vi "Dashboard Main.vi"() -> ()   [LabVIEW 2017]
uses:
  <vilib>/Utility/miscctls.llb/LVRowAndColumnTypeDef.ctl
  <vilib>/event_ctls.llb/eventvkey.ctl
  <vilib>/Rock Robotics/Network Tables/NT Read Numeric Array.vi
  <vilib>/Rock Robotics/WPI/Dashboard/WPI_DashboardLogging Global.vi
panel:
  in  "Camera Settings Right":T1={"Frame Rate"=30, "Compression"=30, "Size"=1, "DB Camera Config"=FALSE} {"Frame Rate" scale=1.0..30.0; "Compression" scale=100.0..-1.0; "Size" items=["640x480", "320x240", "160x120"]}
  in  "Camera Name Right":string(combo)="No Camera Selection"
  out "Camera Info":cluster{"Mbps LED":bool, "Mbps":dbl, "fps":dbl} {"fps" format="%#.1g"; "Mbps" format="%#.1g"}
  in  "Camera Settings":T1={"Frame Rate"=30, "Compression"=30, "Size"=1, "DB Camera Config"=FALSE} {"Frame Rate" scale=1.0..30.0; "Compression" scale=100.0..-1.0; "Size" items=["640x480", "320x240", "160x120"]}
  in  "TCP":refnum<k5>
  in  "Rec Mode":enum32{"Stop", "Record", "Playback"}(radio)
  out "Robot IP":string
  out "Image Message":string="Timeout in Camera Communications"
  in  "Dashboard Tab":T2(tab)
  in  "Select Auto":string(combo)="Select Autonomous ..."
  out "NT Connection":bool
  out "MotorChart R":cluster{"Numeric":dbl, "Numeric":dbl}(graph)
  out "MotorChart L":cluster{"Numeric":dbl, "Numeric":dbl}(graph)
  out "MotorSliders R":cluster{"MotorSlide1":dbl, "MotorSlide2":dbl} {"MotorSlide2" scale=-1.0..1.0 scale format="%#_2e"; "MotorSlide1" scale=-1.0..1.0 scale format="%#_2e"}
  out "MotorSliders L":cluster{"MotorSlide1":dbl, "MotorSlide2":dbl} {"MotorSlide2" scale=-1.0..1.0 scale format="%#_2e"; "MotorSlide1" scale=-1.0..1.0 scale format="%#_2e"}
  out "Gyro":dbl(knob) scale=-360.0..360.0
  out "JS1 Z":dbl(slide) scale=-1.0..1.0 scale format="%#_2e"
  out "JS1 Graph":cluster{"X":dbl, "Y":dbl}[](graph)
  out "JS1 Buttons":T3
  out "JS2 Z":dbl(slide) scale=-1.0..1.0 scale format="%#_2e"
  out "JS2 Graph":cluster{"X":dbl, "Y":dbl}[](graph)
  out "JS2 Buttons":T3
  out "Mode":T4(ring)=enum."Auto Disabled"
  out "Left Position":dbl
  out "Right Position":dbl
  out "Camera Image Right":T5(plugin-control)
  in  "DB/String 9":string
  in  "DB/String 8":string
  in  "DB/String 7":string
  in  "DB/String 6":string
  in  "DB/String 5":string
  in  "DB/String 4":string
  in  "DB/String 3":string
  in  "DB/String 2":string
  in  "DB/String 1":string
  in  "DB/String 0":string
  in  "DB/Slider 0":dbl(slide) scale=0.0..5.0
  in  "DB/Slider 1":dbl(slide) scale=0.0..5.0
  in  "DB/Slider 2":dbl(slide) scale=0.0..5.0
  in  "DB/Slider 3":dbl(slide) scale=0.0..5.0
  out "DB/LED 3":bool
  out "DB/LED 2":bool
  out "DB/LED 1":bool
  out "DB/LED 0":bool
  in  "DB/Button 3":bool
  in  "DB/Button 2":bool
  in  "DB/Button 1":bool
  in  "DB/Button 0":bool caption="New Name"
  out "Tusk Left Output":dbl
  out "Game Specific Data":string
  out "DriveL Position":dbl
  out "DriveR Position":dbl
  out "Tusk Right Position":dbl
  out "Tusk Left Position":dbl
  out "Elbow Position":dbl
  out "Arm Position":dbl
  out "Tusk Right Output":dbl
  in  "Test Slider":dbl(slide) scale=0.0..100.0 scale format="%#_3g"
  in  "On/Off":bool caption="Solenoid"
  in  "Test Name":u16(ring) items=["Select the test to run..."]
  in  "Test Tree":string(tree)
  in  "Motor":cluster{"Value":dbl, "Enable":bool} {"Value" scale=-1.0..1.0 scale format="%#_3g"}
  out "Progress":T6 {"Test Progress" scale=0.0..100.0}
  in  "Rev/Fwd":cluster{"Forward":bool, "Reverse":bool}
  in  "Test Ring":u16(ring) items=["Monochrome", "Color"]
  out "Cmd Status":string
  in  "Execute Command":bool
  in  "Command Params":string[][](table)
  in  "Command Selection":i32(listbox)
  in  "CheckList":i32(listbox)
  out "Tree":string(tree)
  out "Camera Image":T5(plugin-control)
  out "Background":bool
  in  "Camera Name":string(combo)="No Camera Selection"
  # "HW"
  # "HW"
  # "Joysticks"
  # "Drive Motors"
  # "Front"
  # "Right"
  # "Left"
  # "Back"
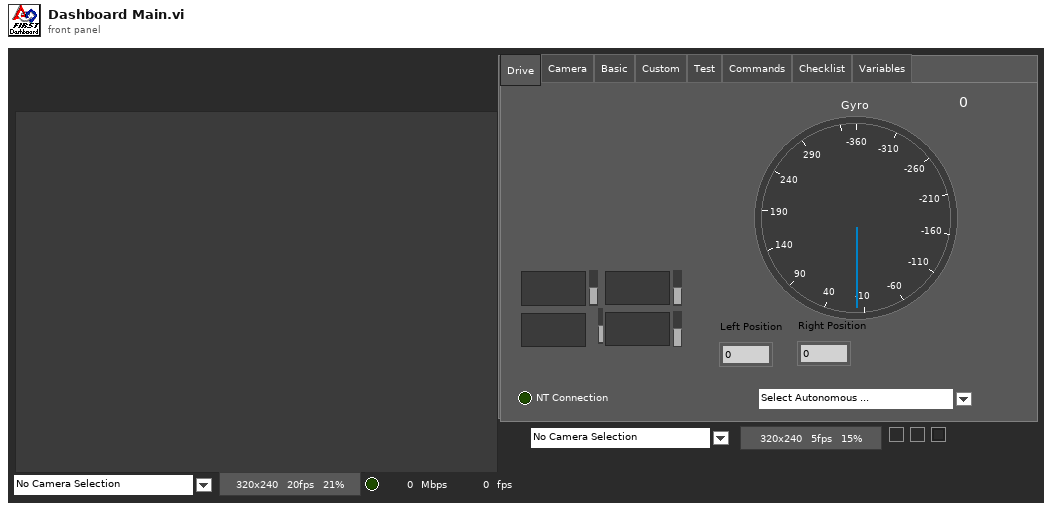
[diagram p1: front panel]
types:
  T1 = cluster{"Frame Rate":i32, "Compression":i32, "Size":u16, "DB Camera Config":bool}
  T2 = enum32{"Drive", "Camera", "Basic", "Custom", "Test", "Commands", "Checklist", "Variables"}
  T3 = cluster{bool, bool, bool, bool, bool, bool, bool, bool, bool, bool, bool, bool}
  T4 = enum8{"Tele-Op Disabled", "Tele-Op Enabled", "Auto Disabled", "Auto Enabled", "Test Disabled", "Test Enabled", "Disconnected", "No Code", "E-Stop"}
  T5 = typedef "IMAQ Image.ctl" = refnum<image>
  T6 = cluster{"Test Progress":u8, "Test Progress Text":string}
  T7 = cluster{"Save Path":path, "Interval (s)":dbl, "Keep":i32}
  T8 = typedef "Image Type" = u32
  T9 = cluster{"IDs":cluster{"RPC field ID":u16, "Unique ID":u16}, "String":string}
  T10 = cluster{"Error Strings":string, "Disable Counts":cluster{u16, u16}, "Rail Faults":cluster{u16, u16, u16}, "Robot IP":string, "DB Mode":u8, "Event Info":cluster{"Name":string, "Type":u8, "Number":u16, "Replay":u8}}
  T11 = cluster{"Storage":cluster{"Disk Free":u64, "RAM Block":u32, "RAM free":u32}, "CPU Utilization":cluster{"CPU % ISR":sgl, "CPU % Time Crit":sgl, "CPU % Timed Str":sgl, "CPU % High":sgl, "CPU % Above":sgl, "CPU % Normal":sgl, "CPU % Low":sgl}, "CAN":cluster{"% Bus Utilization":sgl, "Bus Off Cnt":u32, "TX_FIFO Full Cnt":u32, "Receive Error Cnt":u8, "Transmit Error Cnt":u8}, "HID":cluster{"HID Outputs":u32, "Rumble Low":u16, "Rumble High":u16}[]}
  T12 = cluster{"Status bits":cluster{"Test Mode":bool, "Autonomous":bool, "Enabled":bool, "Code Start":bool, "Brownout":bool, "Reserved 2":bool, "Reserved 3":bool, "E-Stop":bool}, "Code Trace":cluster{"Disabled":bool, "TeleOp":bool, "Auto":bool, "Test":bool}, "Controller Type":enum16{"unknown", "cRIO", "roboRio"}, "Code?":enum16{"unknown", "noCode", "code"}, "Battery V":dbl}
  T13 = cluster{"Control Bits":cluster{"TestMode":bool, "Autonomous":bool, "Enabled":bool, "FMS Present":bool, bool, bool, bool, "E-Stop":bool}, "Team Station ":u8, "Countdown":sgl, "Joystick Values":cluster{"Axes":dbl[], "Buttons":bool[], "POVs":i16[]}[]}
  T14 = cluster{"Axes":dbl[], "Buttons":bool[], "POVs":i16[]}[]
  T15 = cluster{"Axes":dbl[], "Buttons":bool[], "POVs":i16[]}
  T16 = cluster{"Buttons[0]":bool, "Buttons[1]":bool, "Buttons[2]":bool, "Buttons[3]":bool, "Buttons[4]":bool, "Buttons[5]":bool, "Buttons[6]":bool, "Buttons[7]":bool, "Buttons[8]":bool, "Buttons[9]":bool, "Buttons[10]":bool, "Buttons[11]":bool}
  T17 = cluster{"Camera Image":refnum<vi>, "Dashboard Tab":refnum<vi>, "Background":refnum<vi>, "Rec Mode":refnum<vi>, "Test Slider":refnum<vi>, "On/Off ":refnum<vi>, "Test Ring":refnum<vi>, "Rev/Fwd":refnum<vi>, "Test Name":refnum<vi>, "Motor":refnum<vi>, "Progress":refnum<vi>, "CheckList":refnum<vi>, "Tree":refnum<vi>, "Test Tree":refnum<vi>, "Command Params":refnum<vi>, "Command Selection":refnum<vi>, "Execute Command":refnum<vi>, "Cmd Status":refnum<vi>, "Camera Settings":refnum<vi>, "Camera Name":refnum<vi>, "Camera Info":refnum<vi>, "Camera Settings Right":refnum<vi>, "Camera Name Right":refnum<vi>, "Camera Image Right":refnum<vi>}
  T18 = cluster{"Camera Name":string, string, "Saved DB Images Info":cluster{"Save Path":path, "Interval (s)":dbl, "Keep":i32}}
  T19 = cluster{"Camera Name Right":string, string, "Saved DB Images Info":cluster{"Save Path":path, "Interval (s)":dbl, "Keep":i32}}
  T20 = cluster{"Operation":enum16{"Update", "Clear"}, "Color Box":u32}[]
  T21 = typedef "eventvkey.ctl" = enum16{"ASCII", "Enter", "Return", "Shift", "Ctrl", "Alt", "Cmd", "Opt", "Caps", "NumLock", "Clear", "Break", "Up", "Down", "Left", "Right", "Insert", "Delete", "Home", "End", "PageUp", "PageDown", "Escape", "Help", "Pause", "ScrollLock", "F1", "F2", "F3", "F4", "F5", "F6", "F7", "F8", "F9", "F10", "F11", "F12", "F13", "F14", "F15", "F16", "F17", "F18", "F19", "F20", "F21", "F22", "F23", "F24", "Play", "VolumeUp", "VolumeDown", "Mute", "Two Byte Char"}
  T22 = cluster{"Image Size":bool, "Image Type":bool, "Pixel Value":bool, "ROI Information":bool, "Zoom Factor":bool}
  T23 = cluster{"Operation":enum16{"Update", "Clear"}, "Color Box":u32}
  T24 = typedef "LVRowAndColumnTypeDef.ctl" = cluster{"Row":i32, "Column":i32}
  T25 = cluster{"Shift":bool, "Ctrl":bool, "Alt":bool, "Cmd":bool, "Opt":bool}
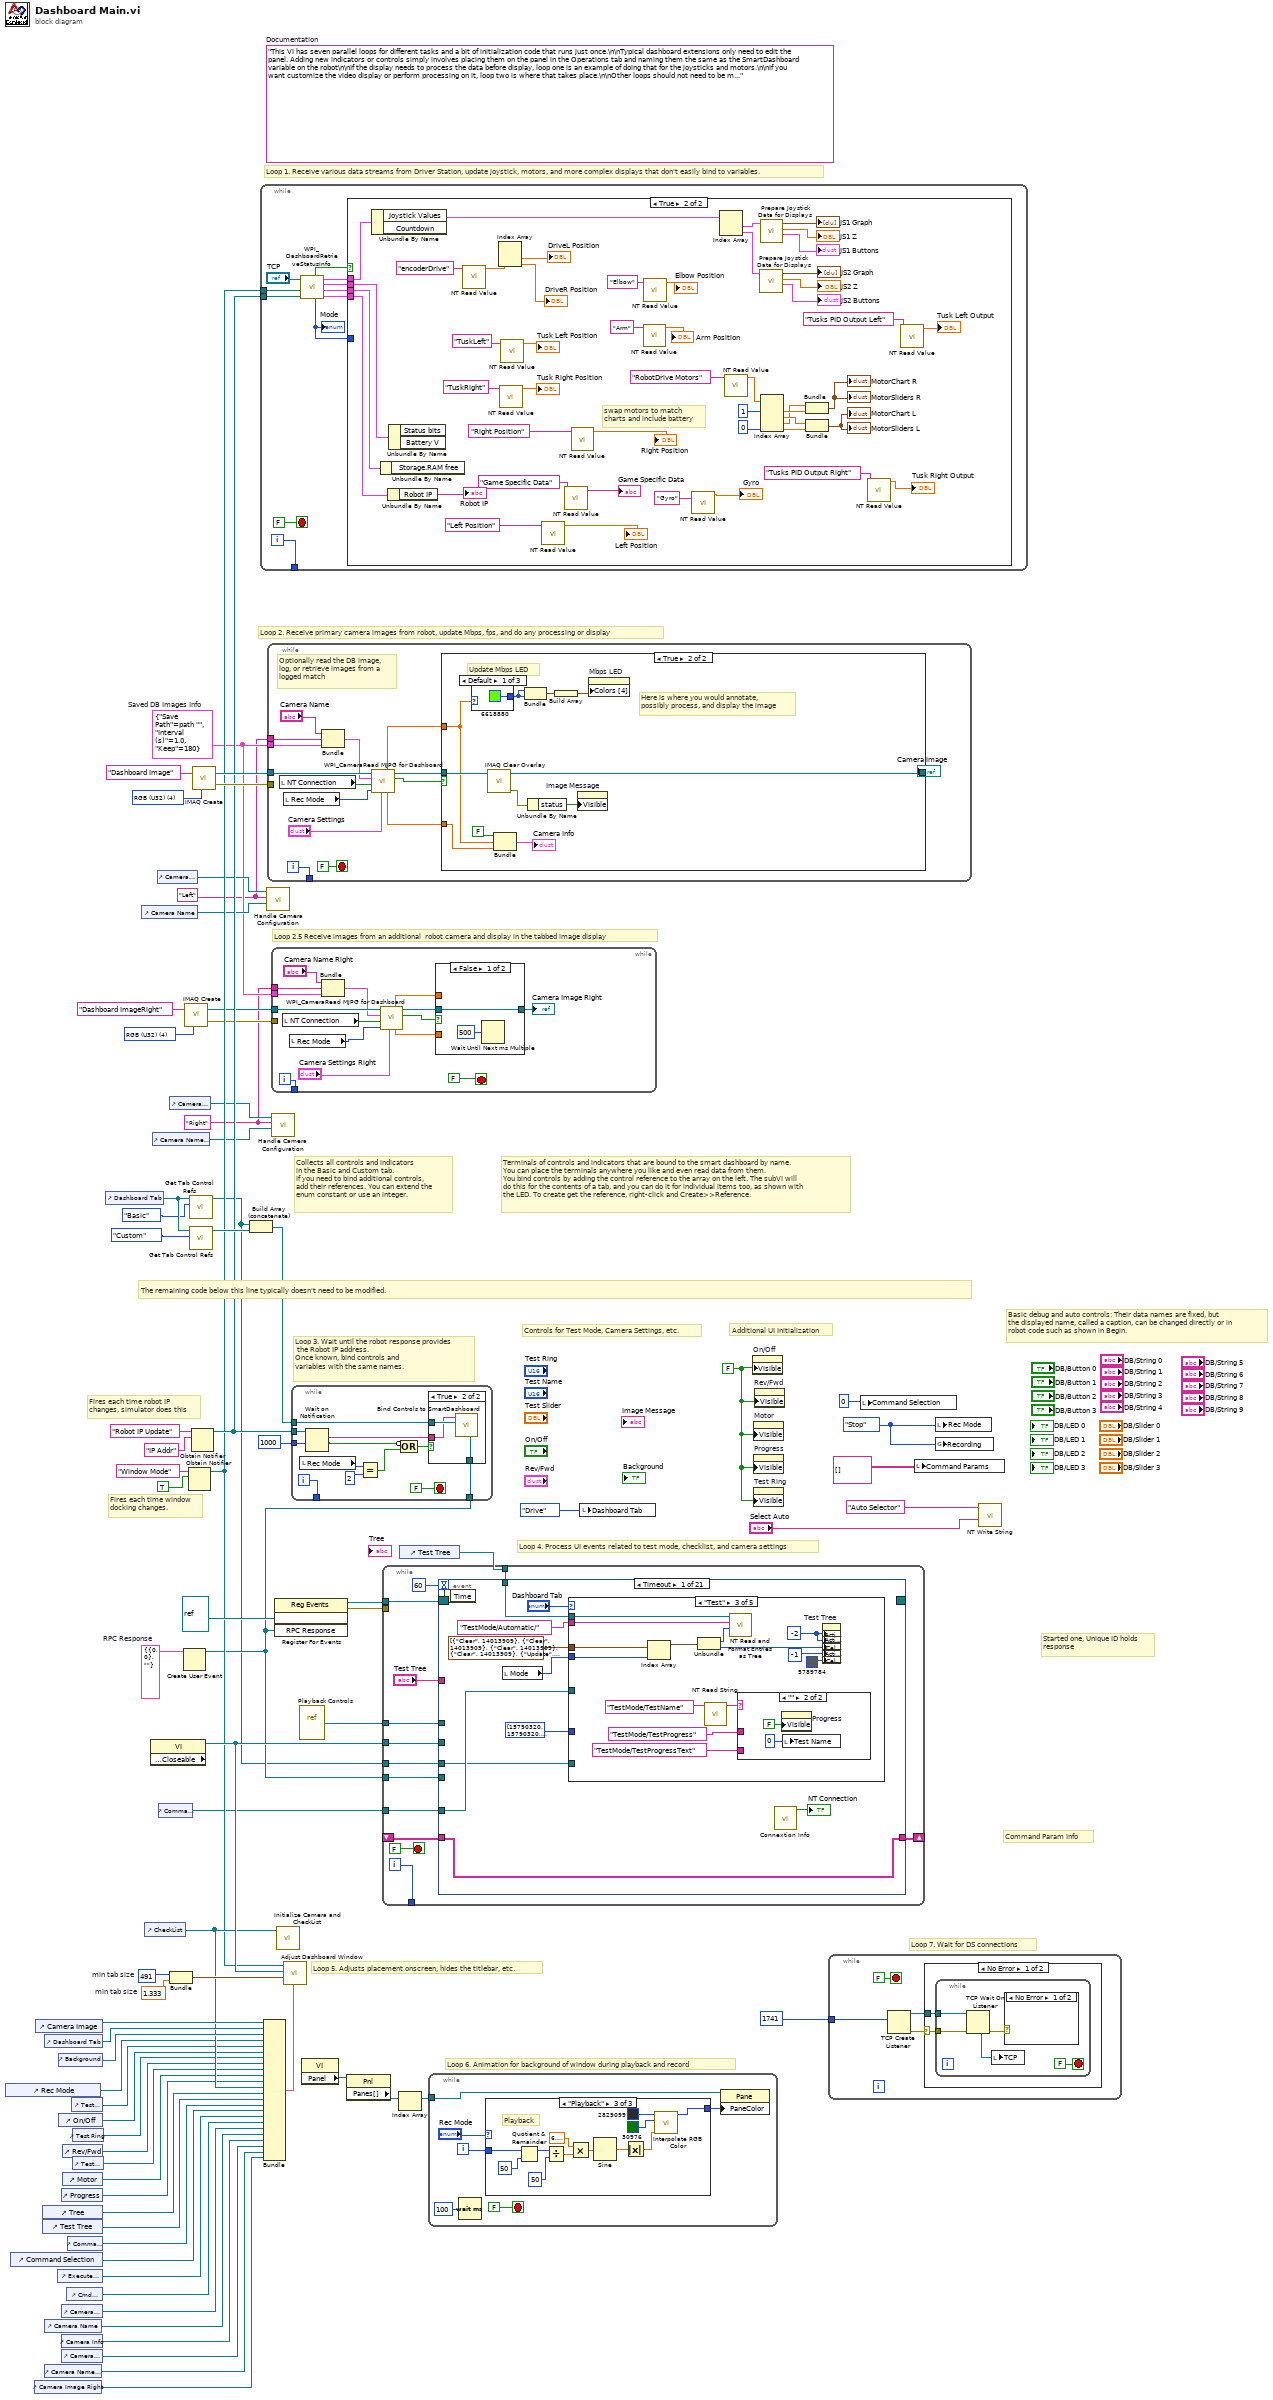
[diagram p0: block diagram]
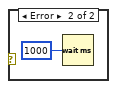
[diagram p3: hidden frame]
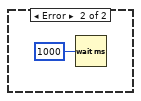
[diagram p4: hidden frame]
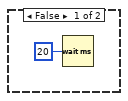
[diagram p5: hidden frame]
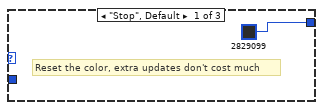
[diagram p6: hidden frame]
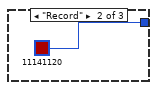
[diagram p7: hidden frame]
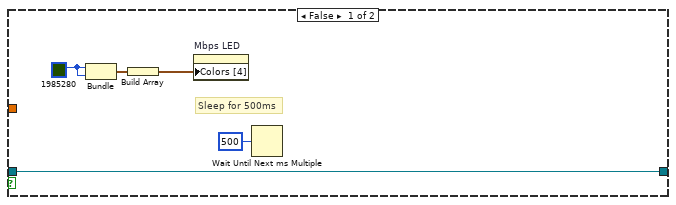
[diagram p9: hidden frame]
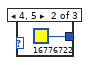
[diagram p10: hidden frame]
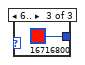
[diagram p11: hidden frame]
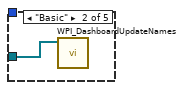
[diagram p13: hidden frame]
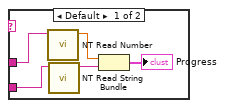
[diagram p14: hidden frame]
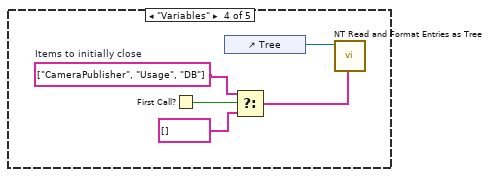
[diagram p15: hidden frame]
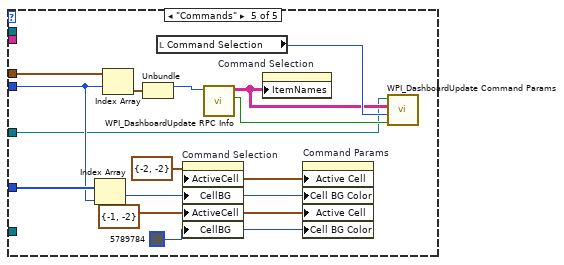
[diagram p16: hidden frame]
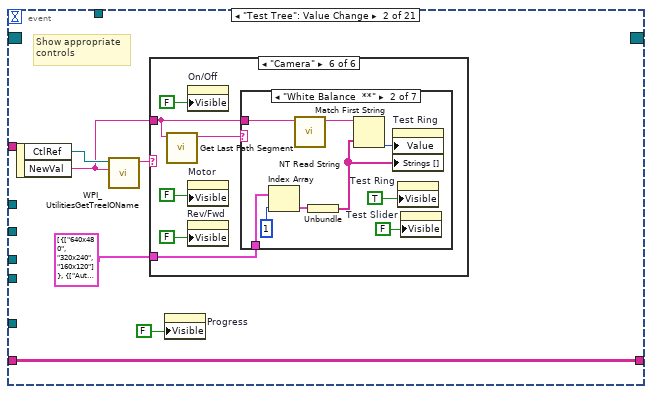
[diagram p17: hidden frame]
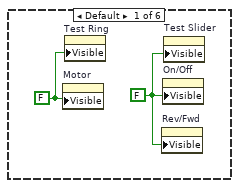
[diagram p18: hidden frame]
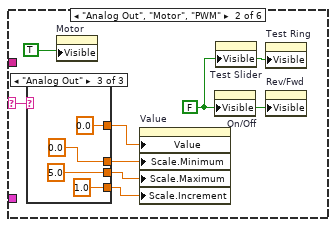
[diagram p19: hidden frame]
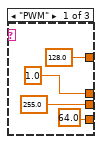
[diagram p20: hidden frame]
diagram:
  w3 = T7 {"Save Path"=path "", "Interval (s)"=1.0, "Keep"=180}  # Saved DB Images Info
  w2 = "Right"
  w1 = "Left"
  w13 = T8 4 items=["Grayscale (U8)", "Grayscale (I16)", "Grayscale (SGL)", "Complex (CSG)", "RGB (U32)", "HSL (U32)", "RGB (U64)"] ("Image Type")
  w29 = T9 {"IDs"={"RPC field ID"=0, "Unique ID"=0}, "String"=""}  # RPC Response
  w52 = 491  # min tab size
  w51 = 1.333  # min tab size
  w59 = enum32{"Stop", "Record", "Playback"}."Stop" ("Rec Mode")
  w36 = FALSE ("Visible")
  (unwired) "This VI has seven parallel loops for different tasks and a bit of initialization code that runs just once.\n\nTypical dashboard extensions only need to edit the panel. Adding new indicators or controls simply involves placing them on the panel in the Operations tab and naming them the same as the SmartDashboard variable on the robot\n\nIf the display needs to process the data before display, loop one is an example of doing that for the joysticks and motors.\n\nIf you want customize the video display or perform processing on it, loop two is where that takes place.\n\nOther loops should not need to be modified. They are pretty standard, and document the task they perform."  # Documentation
  w76 = T8 4 items=["Grayscale (U8)", "Grayscale (I16)", "Grayscale (SGL)", "Complex (CSG)", "RGB (U32)", "HSL (U32)", "RGB (U64)"] ("Image Type")
  # "Loop 2.5 Receive images from an additional  robot camera and display in the tabbed image display"
  # "Command Param Info"
  # "Started one, Unique ID holds\nresponse"
  # "Loop 7. Wait for DS connections"
  # "Basic debug and auto controls: Their data names are fixed, but\nthe displayed name, called a caption, can be changed directly or in\nrobot code such as shown in Begin."
  # "Controls for Test Mode, Camera Settings, etc."
  # "Additional UI Initialization"
  # "Loop 6. Animation for background of window during playback and record"
  # "Fires each time robot IP\nchanges, simulator does this"
  # "Fires each time window\ndocking changes."
  # "Collects all controls and indicators\nin the Basic and Custom tab.\nIf you need to bind additional controls,\nadd their references. You can extend the\nenum constant or use an integer."
  # "The remaining code below this line typically doesn't need to be modified."
  # "Loop 4. Process UI events related to test mode, checklist, and camera settings"
  # "Terminals of controls and indicators that are bound to the smart dashboard by name.\nYou can place the terminals anywhere you like and even read data from them.\nYou bind controls by adding the control reference to the array on the left. The subVI will\ndo this for the contents of a tab, and you can do it for individual items too, as shown with\nthe LED. To create get the reference, right-click and Create>>Reference."
  # "Loop 3. Wait until the robot response provides\n the Robot IP address.\nOnce known, bind controls and\nvariables with the same names."
  # "Loop 5. Adjusts placement onscreen, hides the titlebar, etc."
  # "Loop 1. Receive various data streams from Driver Station, update joystick, motors, and more complex displays that don't easily bind to variables."
  # "Loop 2. Receive primary camera images from robot, update Mbps, fps, and do any processing or display"
  n1 = control-ref of="Rec Mode"() -> (w42:refnum<vi>)
  n2 = control-ref of="Command Selection"() -> (w28:refnum<vi>)
  n3 = control-ref of="Camera Image Right"() -> (w6:refnum<vi>)
  n4 = control-ref of="Camera Image"() -> (w54:refnum<vi>)
  n5 = control-ref of="Tree"() -> (w46:refnum<vi>)
  n6 = control-ref of="Test Tree"() -> (w45:refnum<vi>)
  n7 = control-ref of="Dashboard Tab"() -> (w53:refnum<vi>)
  n8 = control-ref of="Camera Name"() -> (w19:refnum<vi>)
  n9 = control-ref of="Camera Name Right"() -> (w7:refnum<vi>)
  n10 = control-ref of="Execute Command"() -> (w30:refnum<vi>)
  n11 = control-ref of="Background"() -> (w49:refnum<vi>)
  n12 = control-ref of="On/Off"() -> (w40:refnum<vi>)
  n13 = control-ref of="Progress"() -> (w37:refnum<vi>)
  n14 = control-ref of="Camera Settings"() -> (w20:refnum<vi>)
  n15 = control-ref of="Camera Info"() -> (w18:refnum<vi>)
  n16 = control-ref of="Camera Settings Right"() -> (w8:refnum<vi>)
  n17 = control-ref of="Rev/Fwd"() -> (w38:refnum<vi>)
  n18 = control-ref of="Motor"() -> (w43:refnum<vi>)
  n19 = control-ref of="Cmd Status"() -> (w24:refnum<vi>)
  n20 = control-ref of="Command Params"() -> (w31:refnum<vi>)
  n21 = control-ref of="Test Slider"() -> (w41:refnum<vi>)
  n22 = control-ref of="Test Ring"() -> (w39:refnum<vi>)
  n23 = control-ref of="Test Name"() -> (w44:refnum<vi>)
  n24 = control-ref of="Dashboard Tab"() -> (w57:refnum<vi>)
  n25 = control-ref of="Camera Name"() -> (w21:refnum<vi>)
  n26 = control-ref of="CheckList"() -> (w47:refnum<vi>)
  n27 = property class="VI" props=["Front Panel.Closeable"]() -> (reference out=w58:refnum<vi>)  [unwired: 2 in, 2 out]
  n28 = control-ref of="Camera Name Right"() -> (w9:refnum<vi>)
  n29 = control-ref of="Camera Settings"() -> (w22:refnum<vi>)
  n30 = control-ref of="Command Params"() -> (w23:refnum<vi>)
  n31 = control-ref of="Camera Settings Right"() -> (w10:refnum<vi>)
  n32 = Bundle("min tab size"=w52, "min tab size"=w51) -> (w50:cluster{"min tab size":i32, "min tab size":dbl})  [unwired: 1 in]
  n33 = Create User Event(user event datatype=w29) -> (user event=w25:refnum<user-event>)  [unwired: 1 in, 1 out]
  n34 = call "IMAQ Create"("Image Name"="Dashboard ImageRight", "Image Type"=w13) -> ("New Image"=w12:T5, "error out"=w11:errorcluster)  [unwired: 2 in, 1 out]
  n35 = Obtain Notifier(name (unnamed)="Window Mode", notification data type=TRUE) -> (notifier out=w34:refnum<notifier>)  [unwired: 2 in, 2 out]
  n36 = call <vilib>:"Get Tab Control Refs.vi"("Page Index"=T2."Basic" ("Dashboard Tab"), "TabControl in"=w57) -> ("ControlsOnPage"=w17:refnum<vi>[])  [unwired: 9 in]
  n37 = call <vilib>:"Get Tab Control Refs.vi"("Page Index"=T2."Custom" ("Dashboard Tab"), "TabControl in"=w57) -> ("ControlsOnPage"=w56:refnum<vi>[])  [unwired: 9 in]
  n38 = Obtain Notifier(name (unnamed)="Robot IP Update", notification data type="IP Addr" ("name (unnamed)")) -> (notifier out=w35:refnum<notifier>)  [unwired: 2 in, 2 out]
  n39 = call "IMAQ Create"("Image Name"="Dashboard Image", "Image Type"=w76) -> ("New Image"=w74:T5, "error out"=w73:errorcluster)  [unwired: 2 in, 1 out]
  n40 = Build Array (concatenate)(w17, w56) -> (w55:refnum<vi>[])
  n41 = while {
    tunnel: [w86] -> _
    tunnel: w35 -> [w80]
    tunnel: w34 -> [w77]
    i -> [w86]
    stop <- FALSE stop-if-true
    n42 = call <vilib>:"WPI_DashboardRetrieveStatusInfo.vi"("Binding Refnum"=w80, "Window Mode Notifier"=w77, "TCP Cnx"="TCP") -> ("Power and Errors"=w81:T10, "Robot Metrics"=w84:T11, "Status Info"=w85:T12, "Control Info"=w82:T13, "Robot Mode"=w79:T4, "Process?"=w83:bool)  [unwired: 3 in]
    "Mode" <- w79
    n43 = case shown="True" w83 {
      tunnel: w85 -> [_ w136]
      tunnel: w84 -> [_ w135]
      tunnel: w82 -> [_ w134]
      tunnel: w81 -> [_ w133]
      tunnel: w79 -> [_ _]
      frame False {
        n44 = Wait (ms)(milliseconds to wait=u32 20) -> ()  [unwired: 1 out]
      }
      frame True {
        # "swap motors to match\ncharts and include battery"
        n45 = Unbundle By Name(w134) -> ("Joystick Values"=w124:T14)  [unwired: 1 out]
        n46 = Unbundle By Name(w135) -> ()  [unwired: 1 out]
        n47 = Unbundle By Name(w133) -> ("Robot IP"=→"Robot IP":string)
        n48 = Unbundle By Name(w136) -> ()  [unwired: 2 out]
        n49 = call-poly <vilib>:"NT Read Value.vi"("Name"="encoderDrive") -> ("Numeric Array"=w99:dbl[])  [unwired: 9 in, 1 out]
        n50 = Index Array(array=w99) -> (element #1=→"DriveL Position":dbl, element #2=→"DriveR Position":dbl)  [unwired: 2 in]
        n51 = call-poly <vilib>:"NT Read Value.vi"("Name"="TuskRight") -> ("Numeric"=→"Tusk Right Position":dbl)  [unwired: 9 in, 1 out]
        n52 = call-poly <vilib>:"NT Read Value.vi"("Name"="TuskLeft") -> ("Numeric"=→"Tusk Left Position":dbl)  [unwired: 9 in, 1 out]
        n53 = call-poly <vilib>:"NT Read Value.vi"("Name"="Left Position") -> ("Numeric"=→"Left Position":dbl)  [unwired: 9 in, 1 out]
        n54 = call-poly <vilib>:"NT Read Value.vi"("Name"="Game Specific Data") -> ("String"=→"Game Specific Data":string)  [unwired: 9 in, 1 out]
        n55 = call-poly <vilib>:"NT Read Value.vi"("Name"="Right Position") -> ("Numeric"=→"Right Position":dbl)  [unwired: 9 in, 1 out]
        n56 = call-poly <vilib>:"NT Read Value.vi"("Name"="Arm") -> ("Numeric"=→"Arm Position":dbl)  [unwired: 9 in, 1 out]
        n57 = call-poly <vilib>:"NT Read Value.vi"("Name"="Elbow") -> ("Numeric"=→"Elbow Position":dbl)  [unwired: 9 in, 1 out]
        n58 = call-poly <vilib>:"NT Read Value.vi"("Name"="Gyro") -> ("Numeric"=→"Gyro":dbl)  [unwired: 9 in, 1 out]
        n59 = Index Array(array=w124) -> (element #1=w123:T15, element #2=w119:T15)  [unwired: 2 in]
        n60 = call-poly <vilib>:"NT Read Value.vi"("Name"="RobotDrive Motors") -> ("Numeric Array"=w114:dbl[])  [unwired: 9 in, 1 out]
        n61 = call "Prepare Joystick Data for Displays.vi"("Joystick Values"=w119) -> ("Buttons"=→"JS2 Buttons":T16, "Z Axis"=→"JS2 Z":dbl, "Cartesian Data"=→"JS2 Graph":cluster{"X axis":dbl, "X axis":dbl}[])  [unwired: 8 in]
        n62 = call "Prepare Joystick Data for Displays.vi"("Joystick Values"=w123) -> ("Buttons"=→"JS1 Buttons":T16, "Z Axis"=→"JS1 Z":dbl, "Cartesian Data"=→"JS1 Graph":cluster{"X axis":dbl, "X axis":dbl}[])  [unwired: 8 in]
        n63 = Index Array(array=w114, index #1=1, index #4=0) -> (element #1=w128:dbl, element #2=w129:dbl, element #3=w127:dbl, element #4=w132:dbl)  [unwired: 2 in]
        n64 = Bundle("Numeric"=w127, "Numeric"=w128) -> (→"MotorChart R" →"MotorSliders R":cluster{"Numeric":dbl, "Numeric":dbl})  [unwired: 1 in]
        n65 = Bundle("Numeric"=w129, "Numeric"=w132) -> (→"MotorChart L" →"MotorSliders L":cluster{"Numeric":dbl, "Numeric":dbl})  [unwired: 1 in]
        n66 = call-poly <vilib>:"NT Read Value.vi"("Name"="Tusks PID Output Right") -> ("Numeric"=→"Tusk Right Output":dbl)  [unwired: 9 in, 1 out]
        n67 = call-poly <vilib>:"NT Read Value.vi"("Name"="Tusks PID Output Left") -> ("Numeric"=→"Tusk Left Output":dbl)  [unwired: 9 in, 1 out]
      }
    }
  }
  n68 = Bundle("Camera Image"=w54, "Dashboard Tab"=w53, "Background"=w49, "Rec Mode"=w42, "Test Slider"=w41, "On/Off"=w40, "Test Ring"=w39, "Rev/Fwd"=w38, "Test Name"=w44, "Motor"=w43, "Progress"=w37, "CheckList"=w47, "Tree"=w46, "Test Tree"=w45, "Command Params"=w31, "Command Selection"=w28, "Execute Command"=w30, "Cmd Status"=w24, "Camera Settings"=w20, "Camera Name"=w19, "Camera Info"=w18, "Camera Settings Right"=w8, "Camera Name Right"=w7, "Camera Image Right"=w6) -> (w48:T17)  [unwired: 1 in]
  n69 = call "Handle Camera Configuration.vi"("CameraNameRef"=w21, "Display Name"=w1, "ClusterRef"=w22) -> ()  [unwired: 9 in]
  n70 = while {
    tunnel: w74 -> [w149]
    tunnel: w73 -> [_]
    tunnel: [w150] -> _
    tunnel: w3 -> [w140]
    tunnel: w1 -> [w137]
    i -> [w150]
    stop <- FALSE stop-if-true
    # "Optionally read the DB image,\nlog, or retrieve images from a\nlogged match"
    n71 = local read "NT Connection"() -> (w141:bool)
    n72 = local read "Rec Mode"() -> (w145:enum32{"Stop", "Record", "Playback"})
    n73 = Bundle("Camera Name"="Camera Name", w137, "Saved DB Images Info"=w140) -> (w139:T18)  [unwired: 1 in]
    n74 = call <vilib>:"WPI_CameraRead MJPG for Dashboard.vi"("Camera Settings"="Camera Settings", "Rec Mode"=w145, "NT Connection"=w141, "Capture Info"=w139, "Refnum in"=w149) -> ("Active"=w147:bool, "Refnum out"=w148:T5, "FPS"=w146:dbl, "Bandwidth (Mbps)"=w144:dbl)  [unwired: 3 in]
    n75 = case shown="True" w147 {
      tunnel: w148 -> [w152 w163]
      tunnel: w144 -> [_ w160]
      tunnel: w146 -> [_ w161]
      tunnel: [w152 w157] -> w142
      frame False {
        w154 = u32 1985280 ("Color Box")
        # "Sleep for 500ms"
        n76 = Bundle("Color Box"=w154, "Color Box"=w154) -> (w155:cluster{"Color Box":u32, "Color Box":u32})  [unwired: 1 out]
        n77 = Build Array(w155) -> (w153:cluster{"Color Box":u32, "Color Box":u32}[])
        n78 = property on="Mbps LED" class="Bool (strict)"("Colors [4]"=w153) -> ()  [unwired: 2 in, 2 out]
        n79 = Wait Until Next ms Multiple(millisecond multiple=u32 500) -> ()  [unwired: 1 out]
      }
      frame True {
        # "Here is where you would annotate,\npossibly process, and display the image"
        # "Update Mbps LED"
        n80 = case shown="Default" w160 {
          tunnel: [u32 6618880 ("Color Box") u32 16776722 ("Color Box") u32 16716800 ("Color Box")] -> w164
          frame Default {
          }
          frame 4, 5 {
          }
          frame 6.. {
          }
        }
        n81 = call "IMAQ Clear Overlay"("Image"=w163) -> ("error out"=w166:errorcluster, "Image Out"=w157:T5)  [unwired: 2 in, 7 out]
        n82 = Bundle(FALSE, "Bandwidth (Mbps)"=w160, "FPS"=w161) -> (→"Camera Info":cluster{bool, "Bandwidth (Mbps)":dbl, "FPS":dbl})  [unwired: 1 in]
        n83 = Bundle("Color Box"=w164, "Color Box"=w164) -> (w165:cluster{"Color Box":u32, "Color Box":u32})  [unwired: 1 out]
        n84 = Unbundle By Name(w166) -> ("status"=w167:bool)
        n85 = Build Array(w165) -> (w162:cluster{"Color Box":u32, "Color Box":u32}[])
        n86 = property on="Image Message" class="Str"("Visible"=w167) -> ()  [unwired: 2 in, 2 out]
        n87 = property on="Mbps LED" class="Bool (strict)"("Colors [4]"=w162) -> ()  [unwired: 2 in, 2 out]
      }
    }
    "Camera Image" <- w142
  }
  n88 = call "Handle Camera Configuration.vi"("CameraNameRef"=w9, "Display Name"=w2, "ClusterRef"=w10) -> ()  [unwired: 9 in]
  n89 = while {
    tunnel: w12 -> [w185]
    tunnel: w11 -> [_]
    tunnel: [w180] -> _
    tunnel: w3 -> [w174]
    tunnel: w2 -> [w171]
    i -> [w180]
    stop <- FALSE stop-if-true
    n90 = local read "NT Connection"() -> (w175:bool)
    n91 = local read "Rec Mode"() -> (w184:enum32{"Stop", "Record", "Playback"})
    n92 = Bundle("Camera Name Right"="Camera Name Right", w171, "Saved DB Images Info"=w174) -> (w173:T19)  [unwired: 1 in]
    n93 = call <vilib>:"WPI_CameraRead MJPG for Dashboard.vi"("Camera Settings"="Camera Settings Right", "Rec Mode"=w184, "NT Connection"=w175, "Capture Info"=w173, "Refnum in"=w185) -> ("Active"=w179:bool, "Refnum out"=w182:T5, "FPS"=w177:dbl, "Bandwidth (Mbps)"=w178:dbl)  [unwired: 3 in]
    n94 = case shown="False" w179 {
      tunnel: w182 -> [w186 w188]
      tunnel: w178 -> [_ _]
      tunnel: w177 -> [_ _]
      tunnel: [w186 w188] -> w176
      frame False {
        n95 = Wait Until Next ms Multiple(millisecond multiple=u32 500) -> ()  [unwired: 1 out]
      }
      frame True {
      }
    }
    "Camera Image Right" <- w176
  }
  n96 = register-events(refnum<vi> refnum, w25) -> (reference out=w63:refnum<event-registration>, error out=w62:errorcluster)  [unwired: 2 in]
  n97 = call "Initialize Camera and CheckList.vi"("ListBox in"=w47) -> ()  [unwired: 11 in]
  n98 = call "Adjust Dashboard Window.vi"("Sizing Refnums"=w48, "Size Constraints"=w50, "VI"=w58, "WIn Mode"=w34) -> ()  [unwired: 8 in]
  n99 = while {
    tunnel: w55 -> [w200]
    tunnel: w35 -> [w198]
    tunnel: [w196] -> _
    tunnel: u32 1000 ("milliseconds to wait") -> [w195]
    tunnel: w25 -> [w189]
    i -> [w196]
    stop <- FALSE stop-if-true
    n100 = local read "Rec Mode"() -> (w191:enum32{"Stop", "Record", "Playback"})
    n101 = Wait on Notification(notifier=w198, timeout in ms (-1)=w195) -> (notification=w197:string, timed out?=w193:bool)  [unwired: 2 in, 2 out]
    n102 = Equal?(x=w191, y=u16 2 ("Rec Mode")) -> (x = y?=w192:bool)
    n103 = Compound Arithmetic op=OR(invert w193, w192) -> (w194:bool)
    n104 = case shown="True" w194 {
      tunnel: w200 -> [_ w203]
      tunnel: w197 -> [_ w202]
      tunnel: w189 -> [_ w201]
      frame False {
      }
      frame True {
        n105 = call <vilib>:"Bind Controls to SmartDashboard.vi"("RPC ref"=w201, "Bound Control Refs"=w203, "Server IP Address"=w202) -> ()  [unwired: 9 in]
      }
    }
  }
  n106 = vi-ref "Playback Controls.vi"() -> (w64:refnum<vi>)
  n107 = property class="VI"() -> ("Panel"=w66:refnum<vi>)  [unwired: 2 in, 2 out]
  n108 = property class="Pnl"(reference=w66) -> ("Panes[]"=w67:refnum<vi>[])  [unwired: 1 in, 2 out]
  n109 = Index Array(array=w67) -> (element=w65:refnum<vi>)  [unwired: 1 in]
  n110 = control-ref of="Test Tree"() -> (w68:refnum<vi>)
  n111 = while {
    tunnel: [w213] -> _
    tunnel: w68 -> [w212]
    tunnel: w64 -> [w211]
    tunnel: w63 -> [w210]
    tunnel: w62 -> [_]
    tunnel: w58 -> [w209]
    tunnel: w25 -> [w208]
    tunnel: w23 -> [w207]
    shift-right: [w206] -> _
    shift-left: _ -> [w205]
    tunnel: w17 -> [w204]
    i -> [w213]
    stop <- FALSE stop-if-true
    n112 = event shown="[0] Timeout" {
      selector: w210 -> [_ _ _ _ _ _ _ _ _ _ _ _ _ _ _ _ _ _ _ _ _]
      dyn-events: [_ _ _ _ _ _ _ _ _ _ _ _ _ _ _ _ w473 _ _ _ _] -> _
      timeout: u32 60 ("milliseconds to wait") -> [_ _ _ _ _ _ _ _ _ _ _ _ _ _ _ _ _ _ _ _ _]
      tunnel: w212 -> [w225 _ _ _ _ _ _ _ _ _ _ _ _ _ _ _ _ _ _ _ _]
      tunnel: "Test Tree" -> [_ _ _ _ _ _ _ _ _ _ _ w440 w448 w450 w454 w462 _ _ _ _ _]
      tunnel: w211 -> [_ _ _ _ _ _ _ _ _ _ _ _ _ _ _ _ w475 _ w493 _ _]
      tunnel: w209 -> [_ _ _ _ _ _ _ _ _ _ _ _ _ _ _ _ w471 _ _ _ _]
      tunnel: w208 -> [_ _ _ _ _ _ _ _ _ _ _ _ _ _ _ _ w469 _ _ _ _]
      tunnel: w207 -> [w220 _ _ _ _ _ w391 _ _ _ _ _ _ _ _ _ _ _ _ _ _]
      tunnel: [w219 w268 w370 w375 w384 w388 w389 w398 w408 w415 w427 w439 w446 w449 w453 w461 w468 w488 w490 w494 w507] -> w206
      tunnel: w205 -> [w219 w268 w370 w375 w384 w388 w389 _ _ w415 w427 w439 w446 w449 w453 w461 w468 w488 w490 w494 w507]
      tunnel: w204 -> [w217 _ _ _ _ _ _ _ _ _ _ _ _ _ _ _ _ _ _ _ _]
      event Timeout {
        n113 = event-data() -> ()  [unwired: 1 in, 1 out]
        n114 = local read "Mode"() -> (w222:T4)
        n115 = case shown="\"Test\"" "Dashboard Tab" {
          tunnel: w225 -> [_ _ w241 _ _]
          tunnel: "TestMode/Automatic/" ("Name Pattern") -> [_ _ w240 _ _]
          tunnel: T20 [{"Operation"=enum."Clear", "Color Box"=14013909}, {"Operation"=enum."Clear", "Color Box"=14013909}, {"Operation"=enum."Clear", "Color Box"=14013909}, {"Operation"=enum."Clear", "Color Box"=14013909}, {"Operation"=enum."Update", "Color Box"=14013909}, {"Operation"=enum."Update", "Color Box"=16777215}, {"Operation"=enum."Clear", "Color Box"=14013909}, {"Operation"=enum."Clear", "Color Box"=14013909}, {"Operation"=enum."Clear", "Color Box"=14013909}] -> [_ _ w233 _ w261]
          tunnel: w222 -> [_ _ w232 _ w260]
          tunnel: u32[] [15790320, 15790320, 15790320, 15790320, 16777215, 16777215, 15790320, 15790320, 15790320] -> [_ _ _ _ w266]
          tunnel: w220 -> [_ _ _ _ w254]
          tunnel: w217 -> [_ w227 _ _ _]
          frame "Custom", Default {
          }
          frame "Basic" {
            n116 = call <vilib>:"WPI_DashboardUpdateNames.vi"("Controls on Tab"=w227) -> ()  [unwired: 11 in]
          }
          frame "Test" {
            w239 = -2 ("Active Item:Row Number")
            n117 = Index Array(array=w233, index=w232) -> (element=w234:T23)
            n118 = Unbundle(w234) -> ("Operation"=w235:enum16{"Update", "Clear"}, "Color Box"=w236:u32)
            n119 = call <vilib>:"NT Read String.vi"("Name"="TestMode/TestName") -> ("String"=w230:string)  [unwired: 9 in, 1 out]
            n120 = call <vilib>:"NT Read and Format Entries as Tree.vi"("Operation"=w235, "Name Pattern"=w240, "Tree Refnum"=w241) -> ()  [unwired: 7 in, 2 out]
            n121 = case shown="\"\"" w230 {
              tunnel: "TestMode/TestProgress" ("Name") -> [w243 _]
              tunnel: "TestMode/TestProgressText" ("Name") -> [w242 _]
              frame Default {
                n122 = call <vilib>:"NT Read Number.vi"("Name"=w243) -> ("Numeric"=w244:dbl)  [unwired: 9 in, 1 out]
                n123 = call <vilib>:"NT Read String.vi"("Name"=w242) -> ("String"=w245:string)  [unwired: 9 in, 1 out]
                n124 = Bundle("Numeric"=w244, "String"=w245) -> (→"Progress":cluster{"Numeric":dbl, "String":string})  [unwired: 1 in]
              }
              frame "" {
                n125 = property on="Progress" class="Clust (strict)"("Visible"=FALSE) -> ()  [unwired: 2 in, 2 out]
                n126 = local write "Test Name"(u16 0) -> ()
              }
            }
            n127 = property on="Test Tree" class="Tree (strict)"("Active Item Row Number"=w239, "ActiveColNum"=w239, "CellBG"=w236, "Active Item Row Number"=-1 ("Active Item:Row Number"), "CellBG"=u32 5789784 ("Color Box")) -> ()  [unwired: 2 in, 2 out]
          }
          frame "Variables" {
            w251 = string[] ["CameraPublisher", "Usage", "DB"]  # Items to initially close
            n128 = First Call?() -> (First Call?: T/F=w252:bool)
            n129 = control-ref of="Tree"() -> (w253:refnum<vi>)
            n130 = Select(t=w251, s=w252, f=string[] []) -> (s? t:f=w249:string[])
            n131 = call <vilib>:"NT Read and Format Entries as Tree.vi"("Tags to  Close"=w249, "Tree Refnum"=w253) -> ()  [unwired: 8 in, 2 out]
          }
          frame "Commands" {
            w262 = u32 5789784 ("Color Box")
            w263 = T24 {"Row"=-1, "Column"=-2} ("Active Cell:Active Cell")
            w265 = T24 {"Row"=-2, "Column"=-2} ("Active Cell:Active Cell")
            n132 = Index Array(array=w266, index=w260) -> (element=w264:u32)
            n133 = Index Array(array=w261, index=w260) -> (element=w259:T23)
            n134 = Unbundle(w259) -> ("Operation"=w258:enum16{"Update", "Clear"})  [unwired: 1 out]
            n135 = local read "Command Selection"() -> (w257:i32)
            n136 = property on="Command Selection" class="MCListbox (strict)"("ActiveCell"=w265, "CellBG"=w264, "ActiveCell"=w263, "CellBG"=w262) -> ()  [unwired: 2 in, 2 out]
            n137 = call <vilib>:"WPI_DashboardUpdate RPC Info.vi"("Operation"=w258) -> ("update"=w256:bool, "commands"=w255:string[][])  [unwired: 9 in]
            n138 = property on="Command Selection" class="MCListbox (strict)"("ItemNames"=w255) -> ()  [unwired: 2 in, 2 out]
            n139 = property on="Command Params" class="Tbl (strict)"("Active Cell"=w265, "Cell BG Color"=w264, "Active Cell"=w263, "Cell BG Color"=w262) -> ()  [unwired: 2 in, 2 out]
            n140 = call <vilib>:"WPI_DashboardUpdate Command Params.vi"("Update"=w256, "NewVal"=w257, "Commands"=w255, "Param Tbl"=w254) -> ()  [unwired: 7 in, 1 out]
          }
        }
        n141 = call <vilib>:"Connextion Info.vi"() -> ("Connected"=→"NT Connection":bool)  [unwired: 10 in, 1 out]
      }
      event "Test Tree": Value Change {
        # "Show appropriate\ncontrols"
        n142 = event-data() -> ("CtlRef"=w271:refnum<vi>, "NewVal"=w269:string)  [unwired: 1 in]
        n143 = call <vilib>:"WPI_UtilitiesGetTreeIOName.vi"("NewVal"=w269, "TreeControl in"=w271) -> ("I/O Name"=w272:string)  [unwired: 9 in]
        n144 = case shown="\"Camera\"" w272 {
          selector: w272 -> [_ w279 _ w301 w310 _]
          tunnel: w269 -> [_ _ w298 w300 _ w317]
          tunnel: cluster{string[]}[] [{["640x480", "320x240", "160x120"]}, {["Auto", "Fixed indoor", "Fixed outdoor 1", "Fixed outdoor 2", "Fixed fluorescent 1", "Fixed fluorescent 2", "Hold current"]}, {["Auto", "Flicker-free 50 Hz", "Flicker-free 60 Hz", "Hold current"]}, {["None", "Prioritize frame rate", "Prioritize image quality"]}, {["Monochrome", "Color"]}] -> [_ _ _ _ _ w316]
          frame Default {
            w274 = FALSE ("Visible")
            w273 = FALSE ("Visible")
            n145 = property on="Motor" class="Clust (strict)"("Visible"=w273) -> ()  [unwired: 2 in, 2 out]
            n146 = property on="Test Ring" class="Ring (strict)"("Visible"=w273) -> ()  [unwired: 2 in, 2 out]
            n147 = property on="Rev/Fwd" class="Clust (strict)"("Visible"=w274) -> ()  [unwired: 2 in, 2 out]
            n148 = property on="On/Off" class="Bool (strict)"("Visible"=w274) -> ()  [unwired: 2 in, 2 out]
            n149 = property on="Test Slider" class="Slide (strict)"("Visible"=w274) -> ()  [unwired: 2 in, 2 out]
          }
          frame "Analog Out", "Motor", "PWM" {
            w280 = FALSE ("Visible")
            n150 = case shown="\"Analog Out\"" w279 {
              tunnel: [1.0 ("Value") -1.0 ("Value") 0.0 ("Value")] -> w278
              tunnel: [255.0 ("Value") 1.0 ("Value") 5.0 ("Value")] -> w277
              tunnel: [128.0 ("Value") 0.0 ("Value") 0.0 ("Value")] -> w276
              tunnel: [64.0 ("Value") 0.5 ("Value") 1.0 ("Value")] -> w275
              frame "PWM" {
              }
              frame "Motor", Default {
              }
              frame "Analog Out" {
              }
            }
            n151 = property on="Motor" class="Clust (strict)"("Visible"=TRUE) -> ()  [unwired: 2 in, 2 out]
            n152 = property on="Value" class="Slide (strict)"("Value"=w276, "Scale.Minimum"=w278, "Scale.Maximum"=w277, "Scale.Increment"=w275) -> ()  [unwired: 2 in, 2 out]
            n153 = property on="On/Off" class="Bool (strict)"("Visible"=w280) -> ()  [unwired: 2 in, 2 out]
            n154 = property on="Test Slider" class="Slide (strict)"("Visible"=w280) -> ()  [unwired: 2 in, 2 out]
            n155 = property on="Test Ring" class="Ring (strict)"("Visible"=w280) -> ()  [unwired: 2 in, 2 out]
            n156 = property on="Rev/Fwd" class="Clust (strict)"("Visible"=w280) -> ()  [unwired: 2 in, 2 out]
          }
          frame "Servo" {
            w296 = FALSE ("Visible")
            n157 = call <vilib>:"NT Read Number.vi"("Name"=w298) -> ("Numeric"=w297:dbl)  [unwired: 9 in, 1 out]
            n158 = property on="Test Slider" class="Slide (strict)"("Visible"=TRUE, "Scale.Maximum"=170.0 ("Scale.Range:Maximum")) -> ()  [unwired: 2 in, 2 out]
            n159 = local write "Test Slider"(w297) -> ()
            n160 = property on="Motor" class="Clust (strict)"("Visible"=w296) -> ()  [unwired: 2 in, 2 out]
            n161 = property on="Rev/Fwd" class="Clust (strict)"("Visible"=w296) -> ()  [unwired: 2 in, 2 out]
            n162 = property on="On/Off" class="Bool (strict)"("Visible"=w296) -> ()  [unwired: 2 in, 2 out]
            n163 = property on="Test Ring" class="Ring (strict)"("Visible"=w296) -> ()  [unwired: 2 in, 2 out]
          }
          frame "Relay", "Solenoid" {
            w299 = FALSE ("Visible")
            n164 = property on="Motor" class="Clust (strict)"("Visible"=w299) -> ()  [unwired: 2 in, 2 out]
            n165 = property on="Test Slider" class="Slide (strict)"("Visible"=w299) -> ()  [unwired: 2 in, 2 out]
            n166 = Search and Replace String(input string=w300, search string="/Value  **", replace string="/Direction") -> (result string=w306:string)  [unwired: 5 in, 3 out]
            n167 = property on="Test Ring" class="Ring (strict)"("Visible"=w299) -> ()  [unwired: 2 in, 2 out]
            n168 = call <vilib>:"NT Read String.vi"("Name"=w306) -> ("String"=w304:string)  [unwired: 9 in, 1 out]
            n169 = Equal?(x="Both directions", y=w304) -> (x = y?=w302:bool)
            n170 = Not(x=w302) -> (.not. x?=w303:bool)
            n171 = property on="Rev/Fwd" class="Clust (strict)"("Visible"=w302) -> ()  [unwired: 2 in, 2 out]
            n172 = property on="On/Off" class="Bool (strict)"("Visible"=w303, "Caption.Text"=w301) -> ()  [unwired: 2 in, 2 out]
          }
          frame "Compressor", "Digital Out" {
            w309 = FALSE ("Visible")
            # "Get direction and finish"
            n173 = property on="Motor" class="Clust (strict)"("Visible"=w309) -> ()  [unwired: 2 in, 2 out]
            n174 = property on="Test Slider" class="Slide (strict)"("Visible"=w309) -> ()  [unwired: 2 in, 2 out]
            n175 = property on="Test Ring" class="Ring (strict)"("Visible"=w309) -> ()  [unwired: 2 in, 2 out]
            n176 = property on="On/Off" class="Bool (strict)"("Visible"=TRUE, "Caption.Text"=w310) -> ()  [unwired: 2 in, 2 out]
            n177 = property on="Rev/Fwd" class="Clust (strict)"("Visible"=FALSE) -> ()  [unwired: 2 in, 2 out]
          }
          frame "Camera" {
            n178 = call <vilib>:"Get Last Path Segment.vi"("String in"=w317) -> ("String out"=w318:string)  [unwired: 10 in]
            n179 = property on="On/Off" class="Bool (strict)"("Visible"=FALSE) -> ()  [unwired: 2 in, 2 out]
            n180 = property on="Motor" class="Clust (strict)"("Visible"=FALSE) -> ()  [unwired: 2 in, 2 out]
            n181 = property on="Rev/Fwd" class="Clust (strict)"("Visible"=FALSE) -> ()  [unwired: 2 in, 2 out]
            n182 = case shown="\"White Balance  **\"" w318 {
              tunnel: w317 -> [w324 w333 w342 w351 w360 _ w366]
              tunnel: w316 -> [w322 w330 w339 w348 w357 _ _]
              frame "Size  **" {
                n183 = Index Array(array=w322) -> (element=w321:cluster{string[]})  [unwired: 1 in]
                n184 = call <vilib>:"NT Read String.vi"("Name"=w324) -> ("String"=w323:string)  [unwired: 9 in, 1 out]
                n185 = Unbundle(w321) -> (w319:string[])
                n186 = Match First String(2:w319, 3:w323) -> (0:w320:i32)  [unwired: 1 out]
                n187 = property on="Test Ring" class="Ring (strict)"("Value"=w320, "Strings []"=w319) -> ()  [unwired: 2 in, 2 out]
                n188 = property on="Test Ring" class="Ring (strict)"("Visible"=TRUE) -> ()  [unwired: 2 in, 2 out]
                n189 = property on="Test Slider" class="Slide (strict)"("Visible"=FALSE) -> ()  [unwired: 2 in, 2 out]
              }
              frame "White Balance  **" {
                n190 = Index Array(array=w330, index=1) -> (element=w331:cluster{string[]})
                n191 = call <vilib>:"NT Read String.vi"("Name"=w333) -> ("String"=w332:string)  [unwired: 9 in, 1 out]
                n192 = Unbundle(w331) -> (w328:string[])
                n193 = Match First String(2:w328, 3:w332) -> (0:w327:i32)  [unwired: 1 out]
                n194 = property on="Test Ring" class="Ring (strict)"("Value"=w327, "Strings []"=w328) -> ()  [unwired: 2 in, 2 out]
                n195 = property on="Test Ring" class="Ring (strict)"("Visible"=TRUE) -> ()  [unwired: 2 in, 2 out]
                n196 = property on="Test Slider" class="Slide (strict)"("Visible"=FALSE) -> ()  [unwired: 2 in, 2 out]
              }
              frame "Exposure  **" {
                n197 = Index Array(array=w339, index=2) -> (element=w340:cluster{string[]})
                n198 = call <vilib>:"NT Read String.vi"("Name"=w342) -> ("String"=w341:string)  [unwired: 9 in, 1 out]
                n199 = Unbundle(w340) -> (w336:string[])
                n200 = Match First String(2:w336, 3:w341) -> (0:w337:i32)  [unwired: 1 out]
                n201 = property on="Test Ring" class="Ring (strict)"("Value"=w337, "Strings []"=w336) -> ()  [unwired: 2 in, 2 out]
                n202 = property on="Test Ring" class="Ring (strict)"("Visible"=TRUE) -> ()  [unwired: 2 in, 2 out]
                n203 = property on="Test Slider" class="Slide (strict)"("Visible"=FALSE) -> ()  [unwired: 2 in, 2 out]
              }
              frame "Exposure Priority  **" {
                n204 = Index Array(array=w348, index=3) -> (element=w349:cluster{string[]})
                n205 = call <vilib>:"NT Read String.vi"("Name"=w351) -> ("String"=w350:string)  [unwired: 9 in, 1 out]
                n206 = Unbundle(w349) -> (w345:string[])
                n207 = Match First String(2:w345, 3:w350) -> (0:w346:i32)  [unwired: 1 out]
                n208 = property on="Test Ring" class="Ring (strict)"("Value"=w346, "Strings []"=w345) -> ()  [unwired: 2 in, 2 out]
                n209 = property on="Test Ring" class="Ring (strict)"("Visible"=TRUE) -> ()  [unwired: 2 in, 2 out]
                n210 = property on="Test Slider" class="Slide (strict)"("Visible"=FALSE) -> ()  [unwired: 2 in, 2 out]
              }
              frame "Color Enable  **" {
                n211 = Index Array(array=w357, index=4) -> (element=w358:cluster{string[]})
                n212 = call <vilib>:"NT Read String.vi"("Name"=w360) -> ("String"=w359:string)  [unwired: 9 in, 1 out]
                n213 = Unbundle(w358) -> (w354:string[])
                n214 = Match First String(2:w354, 3:w359) -> (0:w355:i32)  [unwired: 1 out]
                n215 = property on="Test Ring" class="Ring (strict)"("Value"=w355, "Strings []"=w354) -> ()  [unwired: 2 in, 2 out]
                n216 = property on="Test Ring" class="Ring (strict)"("Visible"=TRUE) -> ()  [unwired: 2 in, 2 out]
                n217 = property on="Test Slider" class="Slide (strict)"("Visible"=FALSE) -> ()  [unwired: 2 in, 2 out]
              }
              frame Default {
                n218 = property on="Test Ring" class="Ring (strict)"("Visible"=FALSE) -> ()  [unwired: 2 in, 2 out]
                n219 = property on="Test Slider" class="Slide (strict)"("Visible"=FALSE) -> ()  [unwired: 2 in, 2 out]
              }
              frame "Brightness  **", "Color Level  **", "Compression  **", "FPS  **", "Sharpness  **" {
                n220 = call <vilib>:"NT Read Number.vi"("Name"=w366) -> ("Numeric"=w365:dbl)  [unwired: 9 in, 1 out]
                n221 = local write "Test Slider"(w365) -> ()
                n222 = property on="Test Slider" class="Slide (strict)"("Visible"=TRUE, "Scale.Maximum"=100.0 ("Scale.Range:Maximum")) -> ()  [unwired: 2 in, 2 out]
                n223 = property on="Test Ring" class="Ring (strict)"("Visible"=FALSE) -> ()  [unwired: 2 in, 2 out]
              }
            }
          }
        }
        n224 = property on="Progress" class="Clust (strict)"("Visible"=FALSE) -> ()  [unwired: 2 in, 2 out]
      }
      event "Test Name": Mouse Enter {
        # "Populate the ring with the list of tests"
        n225 = event-data() -> ()  [unwired: 1 in, 1 out]
        n226 = call <vilib>:"NT Read String Array.vi"("Name"="TestMode/TestList") -> ("String Array"=w374:string[])  [unwired: 9 in, 1 out]
        n227 = Build Array (concatenate)("Select the test to run...", w374) -> (w373:string[])
        n228 = property on="Test Name" class="Ring (strict)"("Strings []"=w373) -> ()  [unwired: 2 in, 2 out]
      }
      event "Test Name": Value Change {
        w376 = FALSE ("Visible")
        # "Tell the robot the test name to run"
        n229 = event-data() -> ("NewVal"=w380:u16)  [unwired: 1 in]
        n230 = property on="Test Name" class="Ring (strict)"() -> ("Strings []"=w381:string[])  [unwired: 2 in, 2 out]
        n231 = local write "Progress"(T6 {"Test Progress"=0, "Test Progress Text"=""} ("Progress")) -> ()
        n232 = Index Array(array=w381, index=w380) -> (element=w379:string)
        n233 = call <vilib>:"NT Write String.vi"("String"=w379, "Name"="TestMode/TestName") -> ()  [unwired: 9 in, 1 out]
        n234 = property on="Progress" class="Clust (strict)"("Visible"=TRUE) -> ()  [unwired: 2 in, 2 out]
        n235 = property on="Motor" class="Clust (strict)"("Visible"=w376) -> ()  [unwired: 2 in, 2 out]
        n236 = property on="Test Slider" class="Slide (strict)"("Visible"=w376) -> ()  [unwired: 2 in, 2 out]
        n237 = property on="On/Off" class="Bool (strict)"("Visible"=w376) -> ()  [unwired: 2 in, 2 out]
        n238 = property on="Rev/Fwd" class="Clust (strict)"("Visible"=w376) -> ()  [unwired: 2 in, 2 out]
        n239 = property on="Test Ring" class="Ring (strict)"("Visible"=w376) -> ()  [unwired: 2 in, 2 out]
      }
      event "Select Auto": Mouse Enter {
        # "Populate the combo box with the list of autonomous options"
        n240 = event-data() -> ()  [unwired: 1 in, 1 out]
        n241 = call <vilib>:"NT Read String Array.vi"("Name"="Auto List") -> ("String Array"=w383:string[])  [unwired: 9 in, 1 out]
        n242 = property on="Select Auto" class="CmbBox"("Strings[]"=w383) -> ()  [unwired: 2 in, 2 out]
      }
      event "Select Auto": Value Change {
        # "User modified the Auto Selection. Write to NT variable so robot knows."
        n243 = event-data() -> ("NewVal"=w386:string)  [unwired: 1 in]
        n244 = call <vilib>:"NT Write String.vi"("String"=w386, "Name"="Auto Selector") -> ()  [unwired: 9 in, 1 out]
      }
      event "Command Selection": Value Change {
        # "Get the params and show in table"
        n245 = event-data() -> ("NewVal"=w392:i32)  [unwired: 1 in]
        n246 = property on="Command Selection" class="MCListbox (strict)"() -> ("ItemNames"=w390:string[][])  [unwired: 2 in, 2 out]
        n247 = call <vilib>:"WPI_DashboardUpdate Command Params.vi"("NewVal"=w392, "Commands"=w390, "Param Tbl"=w391) -> ()  [unwired: 8 in, 1 out]
      }
      event "Execute Command": Value Change {
        # "Started one, Unique ID holds\nresponse"
        n248 = event-data() -> ()  [unwired: 1 in, 1 out]
        n249 = property on="Command Selection" class="MCListbox (strict)"() -> ("ItemNames"=w403:string[][])  [unwired: 2 in, 2 out]
        n250 = Index Array(array=w403, index (row)="Command Selection", index (col)=0) -> (element=w401:string)
        n251 = call <vilib>:"Invoke Commands.vi"("Command Params"="Command Params", "Function Name"=w401) -> ("Params"=w397:u8, "Started"=w396:bool)  [unwired: 7 in, 1 out]
        n252 = Array Subset(array="Command Params", length (row)=w397) -> (w398:string[][])  [unwired: 3 in]
        n253 = Select(t="Executing" ("Cmd Status"), s=w396, f="" ("Cmd Status")) -> (s? t:f=→"Cmd Status":string)
      }
      event "Command Selection": Double Click {
        n254 = event-data() -> ("Row"=w411:i32)  [unwired: 1 in]
        n255 = property on="Command Selection" class="MCListbox (strict)"() -> ("ItemNames"=w414:string[][])  [unwired: 2 in, 2 out]
        n256 = local read "Command Params"() -> (w410:string[][])
        n257 = Index Array(array=w414, index (row)=w411, index (col)=0) -> (element=w412:string)
        n258 = call <vilib>:"Invoke Commands.vi"("Command Params"=w410, "Function Name"=w412) -> ("Params"=w409:u8, "Started"=w404:bool)  [unwired: 7 in, 1 out]
        n259 = Array Subset(array=w410, length (row)=w409) -> (w408:string[][])  [unwired: 3 in]
        n260 = Select(t="Executing" ("Cmd Status"), s=w404, f="" ("Cmd Status")) -> (s? t:f=w405:string)
        n261 = local write "Cmd Status"(w405) -> ()
      }
      event "CheckList": Double Click {
        # "Shift clears all"
        # "Update symbols on the listbox"
        n262 = event-data() -> ("PlatMods.Shift"=w416:bool, "Row"=w418:i32)  [unwired: 1 in]
        n263 = case shown="True" w416 {
          tunnel: w418 -> [w422 _]
          tunnel: 1 -> [w421 _]
          frame False {
            n264 = property on="CheckList" class="LstBox (strict)"() -> ("Item Symbols"=w420:i32[])  [unwired: 2 in, 2 out]
            n265 = Replace Array Subset(array=w420, new element=w421, index=w422) -> (w419:i32[])
            n266 = property on="CheckList" class="LstBox (strict)"("Item Symbols"=w419) -> ()  [unwired: 2 in, 2 out]
          }
          frame True {
            w423 = 0 ("Top Row")
            n267 = property on="CheckList" class="LstBox (strict)"() -> ("Number of Rows"=w425:u32)  [unwired: 2 in, 2 out]
            n268 = Initialize Array(0, w425) -> (w424:i32[])
            n269 = property on="CheckList" class="LstBox (strict)"("Top Row"=w423, "Value"=w423, "Item Symbols"=w424) -> ()  [unwired: 2 in, 2 out]
          }
        }
      }
      event "CheckList": Key Down {
        # "Update symbols on the listbox\nLeft and right keys check and uncheck"
        n270 = event-data() -> ("VKey"=w429:T21)  [unwired: 1 in]
        n271 = case shown="\"Left\", \"Right\"" w429 {
          selector: w429 -> [w434 _]
          tunnel: eventvkey."Left" ("VKey") -> [w432 _]
          frame "Left", "Right" {
            n272 = Equal?(x=w432, y=w434) -> (x = y?=w433:bool)
            n273 = Select(t=0, s=w433, f=1) -> (s? t:f=w435:i32)
            n274 = property on="CheckList" class="LstBox (strict)"() -> ("Item Symbols"=w438:i32[])  [unwired: 2 in, 2 out]
            n275 = Replace Array Subset(array=w438, new element=w435, index="CheckList") -> (w437:i32[])
            n276 = property on="CheckList" class="LstBox (strict)"("Item Symbols"=w437) -> ()  [unwired: 2 in, 2 out]
          }
          frame Default {
          }
        }
      }
      event "Motor.Enable": Value Change {
        # "When the test mode otor enable helper is set, update that\ntree row item's value"
        n277 = event-data() -> ("NewVal"=w444:bool)  [unwired: 1 in]
        n278 = Unbundle("Motor") -> ("Value"=w443:dbl)  [unwired: 1 out]
        n279 = Select(t=w443, s=w444, f=0.0) -> (s? t:f=w441:dbl)
        n280 = call <vilib>:"NT Write Number.vi"("Numeric"=w441, "Name"=w440) -> ()  [unwired: 9 in, 1 out]
      }
      event "Test Slider": Value Change {
        # "When the test mode slider helper is set, update that\ntree row item's value"
        n281 = event-data() -> ("NewVal"=w447:dbl)  [unwired: 1 in]
        n282 = call <vilib>:"NT Write Number.vi"("Numeric"=w447, "Name"=w448) -> ()  [unwired: 9 in, 1 out]
      }
      event "On/Off": Value Change {
        # "When the test mode on/off helper value is set, update that\ntree row item's value"
        n283 = event-data() -> ("NewVal"=w452:bool)  [unwired: 1 in]
        n284 = Boolean To (0,1)(Boolean=w452) -> (0, 1=w451:i16)
        n285 = call <vilib>:"NT Write Number.vi"("Numeric"=w451, "Name"=w450) -> ()  [unwired: 9 in, 1 out]
      }
      event "Rev/Fwd": Value Change {
        # "When the test mode helper value for relays is set, update that\ntree row item's value"
        n286 = event-data() -> ("NewVal.Forward"=w460:bool, "NewVal.Reverse"=w459:bool)  [unwired: 1 in]
        n287 = Boolean To (0,1)(Boolean=w460) -> (0, 1=w456:i16)
        n288 = Boolean To (0,1)(Boolean=w459) -> (0, 1=w458:i16)
        n289 = Negate(x=w458) -> (-x=w457:i16)
        n290 = Add(x=w456, y=w457) -> (x+y=w455:i16)
        n291 = call <vilib>:"NT Write Number.vi"("Numeric"=w455, "Name"=w454) -> ()  [unwired: 9 in, 1 out]
      }
      event "Test Ring": Value Change {
        # "When a test mode helper value is selected from the ring,\nset the tree item's variable to the string value"
        n292 = event-data() -> ("NewVal"=w464:u16)  [unwired: 1 in]
        n293 = property on="Test Ring" class="Ring (strict)"() -> ("Strings []"=w465:string[])  [unwired: 2 in, 2 out]
        n294 = Index Array(array=w465, index=w464) -> (element=w463:string)
        n295 = call <vilib>:"NT Write String.vi"("String"=w463, "Name"=w462) -> ()  [unwired: 9 in, 1 out]
      }
      event "Rec Mode": Value Change {
        # "Update globals for recording mode and path to read log from.\nClear when logging and let NetworkTables set path for vision to\nuse."
        n296 = event-data() -> ("NewVal"=w476:enum32{"Stop", "Record", "Playback"})  [unwired: 1 in]
        n297 = global write "WPI_DashboardLogging Global.vi" "Logging Filename"(path "") -> ()
        n298 = global write "WPI_DashboardLogging Global.vi" "Recording"(w476) -> ()
        n299 = case shown="\"Playback\"" w476 {
          tunnel: w475 -> [_ w478 w487]
          tunnel: [_ _ w486] -> w473
          tunnel: [_ _ w485] -> _
          tunnel: w471 -> [_ _ w483]
          tunnel: cluster{i32, i32} {-250, 170} -> [_ _ w482]
          tunnel: [_ _ T22 {"Image Size"=TRUE, "Image Type"=TRUE, "Pixel Value"=TRUE, "ROI Information"=TRUE, "Zoom Factor"=FALSE} ("Image Information Shown:All Elements")] -> w466
          tunnel: [_ _ TRUE ("Zoom Factor")] -> w467
          tunnel: w469 -> [_ _ w479]
          frame Default {
          }
          frame "Stop", "Record" {
            # "Place Window too"
            n300 = invoke class="VI" method="FP.Close"(reference=w478) -> (reference out=w477:refnum<vi>)  [unwired: 2 in, 2 out]
            n301 = invoke class="VI" method="Abort VI"(reference=w477) -> ()  [unwired: 2 in, 3 out]
          }
          frame "Playback" {
            n302 = call "Open Playback Panel.vi"("Offset"=w482, "DB VI Ref"=w483, "Playback in"=w487) -> ("Playback out"=w484:refnum<vi>)  [unwired: 8 in]
            n303 = register-events(w484, w479) -> (reference out=w486:refnum<event-registration>, error out=w485:errorcluster)  [unwired: 2 in]
          }
        }
        n304 = property on="Camera Image Right" class="ImageControl"("Image Information Shown"=w466, "Image Information Visible"=w467) -> ()  [unwired: 2 in, 2 out]
        n305 = property on="Camera Image" class="ImageControl"("Image Information Shown"=w466, "Image Information Visible"=w467) -> ()  [unwired: 2 in, 2 out]
        n306 = call <vilib>:"WPI_DashboardNT Log FieldName Cache.vi"("Operation"=enum16{"Lookup/Add", "Index", "Clear"}."Clear") -> ()  [unwired: 8 in, 3 out]
      }
      event Panel Close {
        w489 = enum32{"Stop", "Record", "Playback"}."Stop" ("Rec Mode")
        # "Playback window has been closed, abort"
        n307 = event-data() -> ()  [unwired: 1 in, 4 out]
        n308 = local write "Rec Mode"(w489) -> ()
        n309 = global write "WPI_DashboardLogging Global.vi" "Recording"(w489) -> ()
      }
      event Panel Close {
        # "Abort playback window and ourself"
        n310 = event-data() -> ()  [unwired: 1 in, 4 out]
        n311 = invoke class="VI" method="FP.Close"(reference=w493) -> (reference out=w492:refnum<vi>)  [unwired: 2 in, 2 out]
        n312 = invoke class="VI" method="Abort VI"(reference=w492) -> (error out=w491:errorcluster)  [unwired: 2 in, 2 out]
        n313 = invoke class="VI" method="Abort VI"(error in=w491) -> ()  [unwired: 2 in, 3 out]
      }
      event User Event {
        n314 = event-data() -> ("IDs"=w500:cluster{"RPC field ID":u16, "Unique ID":u16}, "String"=w499:string)  [unwired: 1 in]
        n315 = Bundle("IDs"=w500, "String"=w499) -> (w498:T9)  [unwired: 1 in]
        n316 = call <vilib>:"Retrieve RPC Response.vi"("RPC Response"=w498) -> ("Output"=w496:string[][])  [unwired: 10 in]
        n317 = Build Array (concatenate)(w494, w496) -> (w495:string[][])
        n318 = local write "Command Params"(w495) -> ()
        n319 = local write "Cmd Status"("" ("Cmd Status")) -> ()
      }
      event "Tree": Double Click {
        n320 = event-data() -> ("PlatMods"=w506:T25, "Tag"=w503:string)  [unwired: 1 in]
        n321 = Unbundle(w506) -> ("Shift"=w505:bool)  [unwired: 4 out]
        n322 = String Subset(string=w503, length (rest)=1 ("length (rest)")) -> (substring=w502:string)  [unwired: 1 in]
        n323 = Not(x=w505) -> (.not. x?=w504:bool)
        n324 = case shown="\"/\"" w502 {
          tunnel: w503 -> [_ w509]
          tunnel: w504 -> [_ w508]
          frame Default {
          }
          frame "/" {
            n325 = call <vilib>:"NT Update Persistence.vi"("Persistence"=w508, "Name"=w509) -> ()  [unwired: 9 in, 1 out]
          }
        }
      }
    }
  }
  n326 = while {
    tunnel: w65 -> [w511]
    i -> [w514]
    stop <- FALSE stop-if-true
    n327 = Wait (ms)(milliseconds to wait=u32 100) -> ()  [unwired: 1 out]
    n328 = case shown="\"Playback\"" "Rec Mode" {
      tunnel: w514 -> [_ _ w529]
      tunnel: [u32 2829099 ("Base Color") u32 11141120 ("Target Color") w518] -> w510
      frame "Stop", Default {
        # "Reset the color, extra updates don't cost much"
      }
      frame "Record" {
      }
      frame "Playback" {
        # "Playback"
        n329 = Quotient & Remainder(x=w529, y=u32 50 ("milliseconds to wait")) -> (x-y*floor(x/y)=w525:u32)  [unwired: 1 out]
        n330 = Divide(x=w525, y=u32 50 ("milliseconds to wait")) -> (x/y=w522:dbl)
        n331 = Multiply(x=6.283185307179586, y=w522) -> (x*y=w527:dbl)
        n332 = Sine(x=w527) -> (sin(x)=w526:dbl)
        n333 = Absolute Value(x=w526) -> (abs(x)=w519:dbl)
        n334 = call "Interpolate RGB Color.vi"("Proportion"=w519, "Target Color"=u32 30976, "Base Color"=u32 2829099) -> ("Result Color"=w518:u32)  [unwired: 8 in]
      }
    }
    n335 = property class="Pane"(reference=w511, "PaneColor"=w510) -> ()  [unwired: 1 in, 2 out]
  }
  n336 = local write "Dashboard Tab"(T2."Drive" ("Dashboard Tab")) -> ()
  n337 = property on="On/Off" class="Bool (strict)"("Visible"=w36) -> ()  [unwired: 2 in, 2 out]
  n338 = property on="Motor" class="Clust (strict)"("Visible"=w36) -> ()  [unwired: 2 in, 2 out]
  n339 = property on="Progress" class="Clust (strict)"("Visible"=w36) -> ()  [unwired: 2 in, 2 out]
  n340 = property on="Test Ring" class="Ring (strict)"("Visible"=w36) -> ()  [unwired: 2 in, 2 out]
  n341 = property on="Rev/Fwd" class="Clust (strict)"("Visible"=w36) -> ()  [unwired: 2 in, 2 out]
  n342 = while {
    tunnel: u16 1741 ("timeout ms (25000)") -> [w531]
    stop <- FALSE stop-if-true
    n343 = TCP Create Listener(10:w531) -> (0:w530:errorcluster, 3:w532:refnum<k5>)  [unwired: 4 in, 1 out]
    n344 = case shown="No Error" w530 {
      selector: w530 -> [w534 _]
      tunnel: w532 -> [w535 _]
      frame No Error {
        n345 = while {
          tunnel: w535 -> [w538]
          tunnel: w534 -> [w537]
          stop <- FALSE stop-if-true
          n346 = TCP Wait On Listener(8:w537, 11:w538) -> (0:w539:errorcluster, 4:w540:refnum<k5>)  [unwired: 2 in, 3 out]
          n347 = local write "TCP"(w540) -> ()
          n348 = case shown="No Error" w539 {
            frame No Error {
            }
            frame Error {
              n349 = Wait (ms)(milliseconds to wait=u32 1000) -> ()  [unwired: 1 out]
            }
          }
        }
      }
      frame Error {
        n350 = Wait (ms)(milliseconds to wait=u32 1000) -> ()  [unwired: 1 out]
      }
    }
  }
  n351 = local write "Command Selection"(u16 0 ("milliseconds to wait")) -> ()
  n352 = local write "Command Params"(string[][] [] ("Command Params")) -> ()
  n353 = global write "WPI_DashboardLogging Global.vi" "Recording"(w59) -> ()
  n354 = local write "Rec Mode"(w59) -> ()
  n355 = call <vilib>:"NT Write String.vi"("String"="Select Auto", "Name"="Auto Selector") -> ()  [unwired: 9 in, 1 out]
